vi "Normaliz4.vi"(4 "data info template":refnum<vi>, 5 "waveform in":waveform(dbl)) -> (2 "waveform out":waveform(dbl))   [LabVIEW 2014]
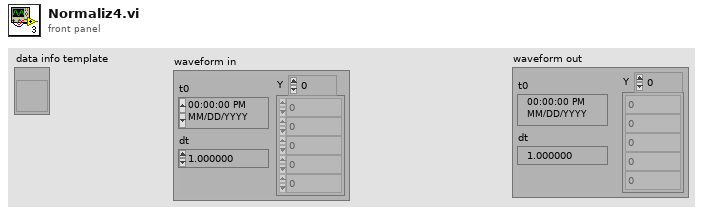
[diagram p1: front panel]
types:
  T1 = cluster{"data path":string, "ADCintercadr_s":dbl, "data info":cluster{"use or not *.info.txt?":i16, "probe name":string, "signal type":string, "Unit":string, "variable":string, "attenuation factor":dbl, "amplification factor":dbl, "extracoef#1":dbl, "extracoef#2":dbl, "U cascade, kV":string, "probe area, cm2":dbl, "plasma, a.m.u.":dbl}, "channel_name":string, "channels_in_file":i32, "LastModified":string}
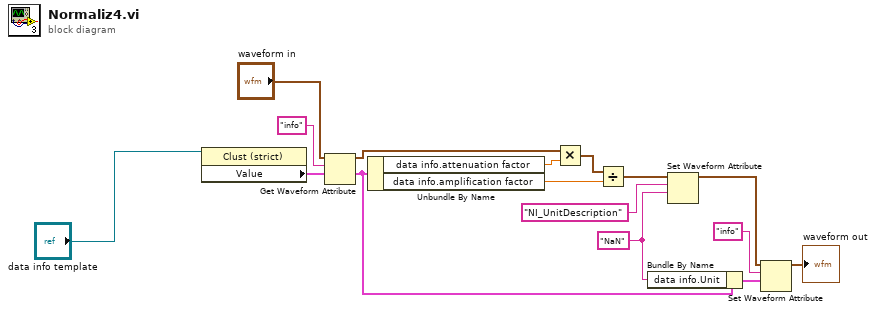
[diagram p0: block diagram]
diagram:
  w5 = "NaN" ("Unit")
  n1 = property class="Clust (strict)"(reference="data info template") -> ("Value"=w16:T1)  [unwired: 1 in, 2 out]
  n2 = Get Waveform Attribute(5:w16, 6:"info" ("name"), 7:"waveform in") -> (1:w6:T1, 3:w14:waveform(dbl))  [unwired: 1 in, 2 out]
  n3 = Unbundle By Name(w6) -> ("data info.attenuation factor"=w10:dbl, "data info.amplification factor"=w11:dbl)
  n4 = Multiply(x=w14, y=w10) -> (x*y=w12:waveform(dbl))
  n5 = Divide(x=w12, y=w11) -> (x/y=w9:waveform(dbl))
  n6 = Bundle By Name(cluster=w6, "data info.Unit"=w5) -> (w4:T1)
  n7 = Set Waveform Attribute(5:w5, 6:"NI_UnitDescription" ("name"), 7:w9) -> (3:w8:waveform(dbl))  [unwired: 1 in, 2 out]
  n8 = Set Waveform Attribute(5:w4, 6:"info" ("name"), 7:w8) -> (3:→"waveform out":waveform(dbl))  [unwired: 1 in, 2 out]
